vi "Add Plugin Group Sections.vi"(8 "error in (no error)":errorcluster, 11 "Item Ref in":T1 format="%.0x") -> (0 "error out":errorcluster, 3 "Item Ref out":T1 format="%.0x")   [LabVIEW 2017, in "DSF System Explorer.lvlib"]
uses:
  DSF System Explorer.lvlib
  <vilib>/NI Veristand/Custom Device API/Custom Device Item Ref.ctl
  DSF Core.lvlibp/Classes/Configuration/Read All Plugin IDs.vi
  Shared/Plugin Page GUID.vi
  <vilib>/NI Veristand/Custom Device API/Set Item Property (String).vi
  <vilib>/NI Veristand/Custom Device API/Custom Device API.lvlib
  DSF Core.lvlibp/Classes/Configuration/Configuration Session.lvclass
  Shared/DSF Shared.lvlib
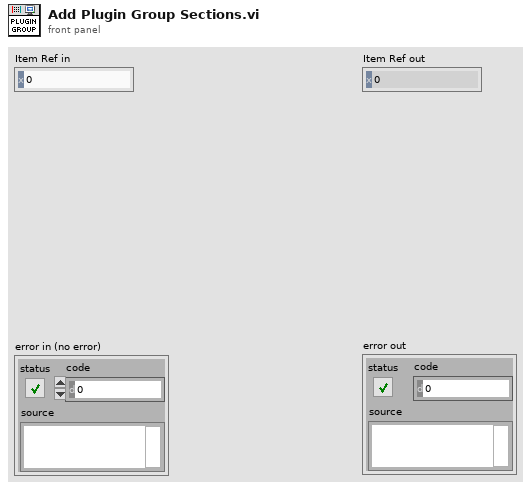
[diagram p1: front panel]
types:
  T1 = typedef "Custom Device API.lvlib/Custom Device Item Ref.ctl" = u64
  T2 = typedef "DSF System Explorer.lvlib/shared data ref.ctl" = refnum<data-value>
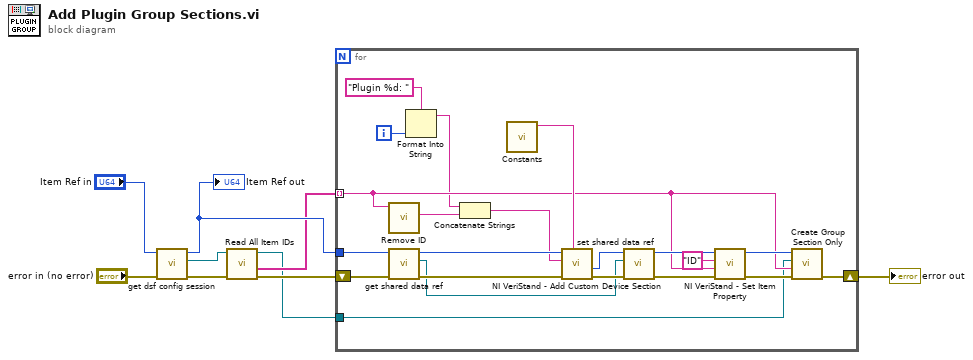
[diagram p0: block diagram]
diagram:
  n1 = call "get dsf config session.vi"("error in (no error)"="error in (no error)", "Item Ref in"="Item Ref in") -> ("error out"=w7:errorcluster, "Configuration Session"=w5:refnum<class "Configuration Session.lvclass">, "Item Ref out"=w4:T1)  [unwired: 7 in]
  "Item Ref out" <- w4
  n2 = call-poly "Read All Item IDs.vi"("error in (no error)"=w7, "Configuration Session in"=w5) -> ("error out"=w9:errorcluster, "Plugin IDs"=w2:string[], "Configuration Session out"=w1:refnum<class "Configuration Session.lvclass">)  [unwired: 7 in]
  n3 = for {
    tunnel: w2 -> [w16] mode=indexing
    tunnel: w4 -> [w28]
    tunnel: w1 -> [w10]
    shift-right: [w30] -> w3
    shift-left: w9 -> [w27]
    i -> [w15]
    n4 = call "Remove ID.vi"("id string"=w16) -> ("name"=w12:string)  [unwired: 8 in, 2 out]
    n5 = call "get shared data ref.vi"("error in (no error)"=w27, "Item Ref in"=w28) -> ("error out"=w25:errorcluster, "shared data ref"=w20:T2, "Item Ref out"=w26:T1)  [unwired: 7 in]
    n6 = Format Into String(format string="Plugin %d: ", w15) -> (resulting string=w13:string)  [unwired: 2 in, 1 out]
    n7 = Concatenate Strings(w13, w12) -> (w11:string)
    n8 = call-poly "Constants.vi"() -> ("Plugin GUID"=w17:string)  [unwired: 11 in]
    n9 = call <vilib>:"NI VeriStand - Add Custom Device Section.vi"("GUID (Default Section)"=w17, "error in (no error)"=w25, "Section Name"=w11, "Parent Ref in"=w26) -> ("error out"=w23:errorcluster, "Section Ptr"=w24:T1)  [unwired: 4 in, 2 out]
    n10 = call "set shared data ref.vi"("error in (no error)"=w23, "shared data ref"=w20, "Node Ptr"=w24) -> ("error out"=w22:errorcluster, "Item Ref out"=w21:T1)  [unwired: 7 in]
    n11 = call-poly <vilib>:"NI VeriStand - Set Item Property.vi"("error in (no error)"=w22, "Value"=w16, "Property Name"="ID", "Item Ref in"=w21) -> ("error out"=w18:errorcluster, "Item Ref out"=w19:T1)  [unwired: 5 in, 1 out]
    n12 = call "Create Group Section Only.vi"("error in (no error)"=w18, "String"=w16, "dsf refnum in"=w10, "Section Ptr"=w19) -> ("error out"=w30:errorcluster)  [unwired: 7 in]
  }
  "error out" <- w3
